vi "Generate XML File.vi"(8 "error in (no error)":errorcluster, 10 "Code Coverage":map{path, dbl}(c390), 11 "Coverage Report in":refnum<class "Coverage Report.lvclass">) -> (0 "error out":errorcluster, 2 "Report Path":path, 3 "Coverage Report out":refnum<class "Coverage Report.lvclass">)   [LabVIEW 2020, in "Coverage Report.lvclass"]
uses:
  Coverage Report.lvclass
  C:/Program Files (x86)/National Instruments/LabVIEW 2020/vi.lib/Astemes/LUnit/Framework/Report Plugin/LUnit Report Plugin.lvclass
  Coverage Report.lvclass/Coverage Report.ctl
  <vilib>/xml/Close Reference(Node).vi
  <vilib>/xml/NI_XML.lvlib
  <resource>/objmgr/DOMUserDefRef.rc
  <vilib>/Astemes/LUnit/Framework/Report Plugin/LUnit Report Plugin.lvclass
  C:/Program Files (x86)/National Instruments/LabVIEW 2020/vi.lib/Astemes/LUnit/Framework/Plugin/LUnit Plugin.lvclass
  C:/git/astemes-lunit-coverage-report/source/Coverage Report/Coverage Report.lvclass
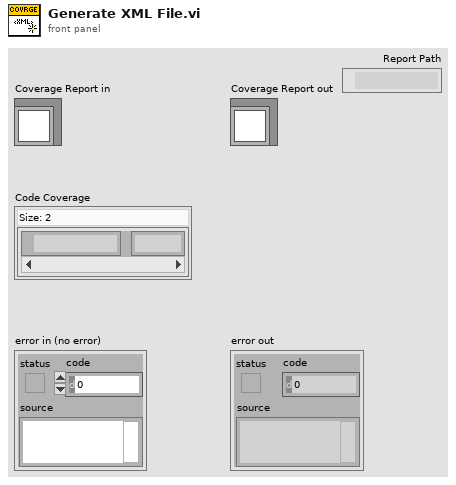
[diagram p1: front panel]
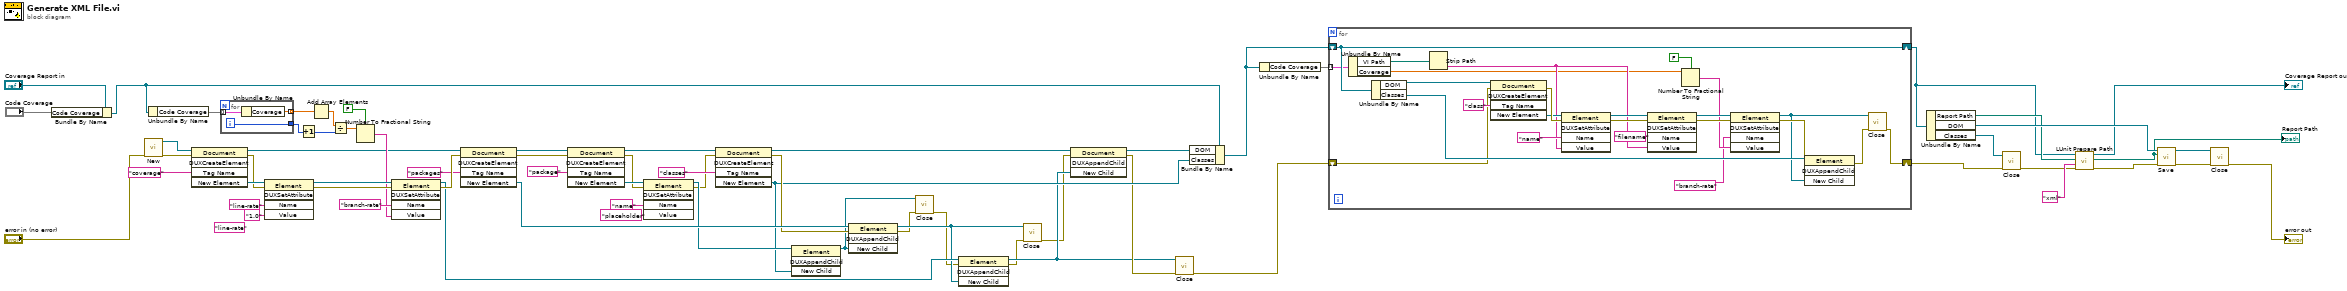
[diagram p0: block diagram]
diagram:
  (unwired) "line-rate" ("Name")
  n1 = Bundle By Name(cluster="Coverage Report in", "Code Coverage"="Code Coverage") -> (w23:refnum<class "Coverage Report.lvclass">)
  n2 = call <vilib>:"New.vi"("error in (no error)"="error in (no error)") -> ("error out"=w65:errorcluster, "DOM document out"=w66:refnum<k20>)  [unwired: 7 in]
  n3 = Unbundle By Name(w23) -> ("Code Coverage"=w22:map{path, dbl})
  n4 = invoke class="Document" method="DUXCreateElement"(reference=w66, error in=w65, "Tag Name"="coverage") -> (reference out=w46:refnum<k20>, error out=w58:errorcluster, "New Element"=w59:refnum<k20>)  [unwired: 2 in, 2 out]
  n5 = for {
    tunnel: w22 -> [w69] mode=indexing
    tunnel: [w68] -> w52 mode=indexing
    tunnel: [w67] -> w50
    i -> [w67]
    n6 = Unbundle By Name(w69) -> ("Coverage"=w68:dbl)
  }
  n7 = invoke class="Element" method="DUXSetAttribute"(reference=w59, error in=w58, "Name"="line-rate", "Value"="1.0") -> (reference out=w55:refnum<k20>, error out=w54:errorcluster)  [unwired: 1 in, 3 out]
  n8 = Increment(x=w50) -> (x+1=w19:i32)
  n9 = Add Array Elements(numeric array=w52) -> (sum=w51:dbl)
  n10 = Divide(x=w51, y=w19) -> (x/y=w49:dbl)
  n11 = Number To Fractional String(use system decimal point (T)=FALSE, number=w49) -> (F-format string=w47:string)  [unwired: 2 in]
  n12 = invoke class="Element" method="DUXSetAttribute"(reference=w55, error in=w54, "Name"="branch-rate", "Value"=w47) -> (reference out=w43:refnum<k20>, error out=w45:errorcluster)  [unwired: 1 in, 3 out]
  n13 = invoke class="Document" method="DUXCreateElement"(reference=w46, error in=w45, "Tag Name"="packages") -> (reference out=w42:refnum<k20>, error out=w40:errorcluster, "New Element"=w35:refnum<k20>)  [unwired: 2 in, 2 out]
  n14 = invoke class="Document" method="DUXCreateElement"(reference=w42, error in=w40, "Tag Name"="package") -> (reference out=w34:refnum<k20>, error out=w37:errorcluster, "New Element"=w38:refnum<k20>)  [unwired: 2 in, 2 out]
  n15 = invoke class="Element" method="DUXSetAttribute"(reference=w38, error in=w37, "Name"="name", "Value"="placeholder") -> (reference out=w31:refnum<k20>, error out=w30:errorcluster)  [unwired: 1 in, 3 out]
  n16 = invoke class="Document" method="DUXCreateElement"(reference=w34, error in=w30, "Tag Name"="classes") -> (reference out=w33:refnum<k20>, error out=w29:errorcluster, "New Element"=w26:refnum<k20>)  [unwired: 2 in, 2 out]
  n17 = invoke class="Element" method="DUXAppendChild"(reference=w31, "New Child"=w26) -> (reference out=w1:refnum<k20>)  [unwired: 2 in, 3 out]
  n18 = invoke class="Element" method="DUXAppendChild"(reference=w35, error in=w29, "New Child"=w1) -> (reference out=w6:refnum<k20>, error out=w3:errorcluster)  [unwired: 1 in, 2 out]
  n19 = call-poly <vilib>:"Close.vi"("error in (no error)"=w3, "node"=w1) -> ("error out"=w2:errorcluster)  [unwired: 7 in]
  n20 = invoke class="Element" method="DUXAppendChild"(reference=w43, error in=w2, "New Child"=w6) -> (reference out=w7:refnum<k20>, error out=w5:errorcluster)  [unwired: 1 in, 2 out]
  n21 = call-poly <vilib>:"Close.vi"("error in (no error)"=w5, "node"=w6) -> ("error out"=w4:errorcluster)  [unwired: 7 in]
  n22 = invoke class="Document" method="DUXAppendChild"(reference=w33, error in=w4, "New Child"=w7) -> (reference out=w27:refnum<k20>, error out=w9:errorcluster)  [unwired: 1 in, 2 out]
  n23 = call-poly <vilib>:"Close.vi"("error in (no error)"=w9, "node"=w7) -> ("error out"=w8:errorcluster)  [unwired: 7 in]
  n24 = Bundle By Name(cluster=w23, "DOM"=w27, "Classes"=w26) -> (w21:refnum<class "Coverage Report.lvclass">)
  n25 = Unbundle By Name(w21) -> ("Code Coverage"=w20:map{path, dbl})
  n26 = for {
    shift-right: [w71] -> w12
    shift-left: w8 -> [w90]
    shift-right: [w88] -> w15
    shift-left: w21 -> [w88]
    tunnel: w20 -> [w87] mode=indexing
    n27 = Unbundle By Name(w87) -> ("VI Path"=w86:path, "Coverage"=w75:dbl)
    n28 = Unbundle By Name(w88) -> ("DOM"=w92:refnum<k20>, "Classes"=w91:refnum<k20>)
    n29 = Strip Path(path=w86) -> (name=w80:string)  [unwired: 1 out]
    n30 = invoke class="Document" method="DUXCreateElement"(reference=w92, error in=w90, "Tag Name"="class") -> (error out=w89:errorcluster, "New Element"=w85:refnum<k20>)  [unwired: 2 in, 3 out]
    n31 = invoke class="Element" method="DUXSetAttribute"(reference=w85, error in=w89, "Name"="name", "Value"=w80) -> (reference out=w83:refnum<k20>, error out=w82:errorcluster)  [unwired: 1 in, 3 out]
    n32 = invoke class="Element" method="DUXSetAttribute"(reference=w83, error in=w82, "Name"="filename", "Value"=w80) -> (reference out=w79:refnum<k20>, error out=w78:errorcluster)  [unwired: 1 in, 3 out]
    n33 = Number To Fractional String(use system decimal point (T)=FALSE, number=w75) -> (F-format string=w74:string)  [unwired: 2 in]
    n34 = invoke class="Element" method="DUXSetAttribute"(reference=w79, error in=w78, "Name"="branch-rate", "Value"=w74) -> (reference out=w70:refnum<k20>, error out=w77:errorcluster)  [unwired: 1 in, 3 out]
    n35 = invoke class="Element" method="DUXAppendChild"(reference=w91, error in=w77, "New Child"=w70) -> (error out=w72:errorcluster)  [unwired: 1 in, 3 out]
    n36 = call-poly <vilib>:"Close.vi"("error in (no error)"=w72, "node"=w70) -> ("error out"=w71:errorcluster)  [unwired: 7 in]
  }
  n37 = Unbundle By Name(w15) -> ("Report Path"=w17:path, "DOM"=w28:refnum<k20>, "Classes"=w10:refnum<k20>)
  n38 = call-poly <vilib>:"Close.vi"("error in (no error)"=w12, "node"=w10) -> ("error out"=w11:errorcluster)  [unwired: 7 in]
  n39 = call <vilib>:"LUnit Prepare Path.vi"("error in (no error)"=w11, "Extenssion"="xml", "File Path in"=w17, "Plugin In"=w15) -> ("error out"=w18:errorcluster, "Modified Path"=w16:path, "Plugin Out"=→"Coverage Report out":refnum<class "Coverage Report.lvclass">)  [unwired: 5 in]
  "Report Path" <- w16
  n40 = call <vilib>:"Save.vi"("error in (no error)"=w18, "XML file path"=w16, "DOM document in"=w28) -> ("error out"=w62:errorcluster, "DOM document out"=w63:refnum<k20>)  [unwired: 6 in, 1 out]
  n41 = call-poly <vilib>:"Close.vi"("error in (no error)"=w62, "node"=w63) -> ("error out"=→"error out":errorcluster)  [unwired: 7 in]
